vi "Auto New Vision.vi"(11 "Run?":bool) -> (2 "Side?":dbl, 3 "Done":bool)   [LabVIEW 2013]
panel:
  out "Particle Measurements (Pixels)":dbl[][](array[numeric]) format="%.2f"
  out "element":dbl
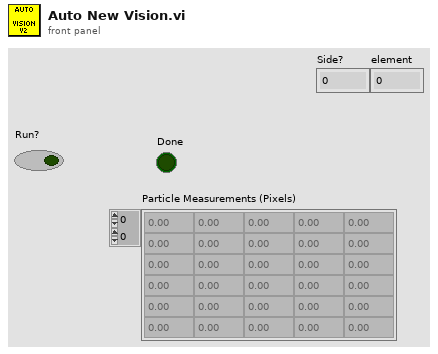
[diagram p1: front panel]
types:
  T1 = typedef "WPI_CameraDevRef.ctl" = cluster{"Camera Address":string, "CameraStatus":errorcluster, "Acquire Image Notifier":refnum<notifier>}
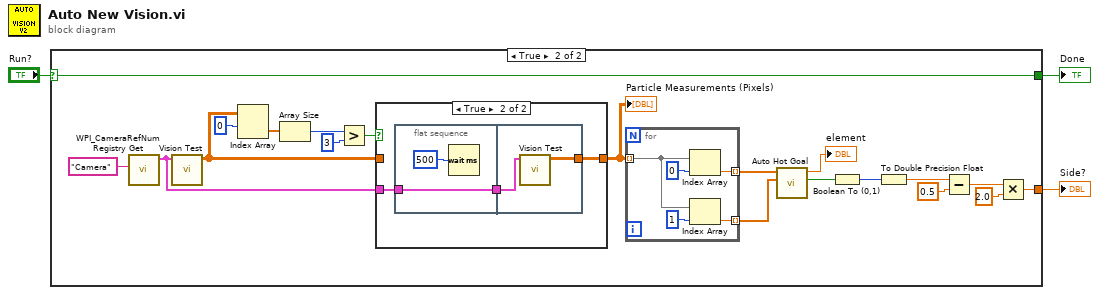
[diagram p0: block diagram]
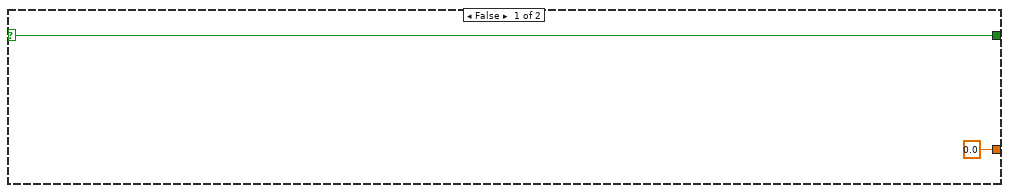
[diagram p2: hidden frame]
diagram:
  n1 = case shown="True" "Run?" {
    selector: "Run?" -> [w5 w25]
    tunnel: [w5 w25] -> w2
    tunnel: [0.0 w15] -> w1
    frame False {
    }
    frame True {
      n2 = call <vilib>:"WPI_CameraRefNum Registry Get.vi"("refnum name"="Camera") -> ("CameraDevRef"=w8:T1)  [unwired: 9 in, 1 out]
      n3 = call "Vision Test.vi"("CameraDevRef"=w8) -> ("Particle Measurements (Pixels)"=w7:dbl[][])  [unwired: 9 in, 1 out]
      n4 = Index Array(array=w7, index (row)=0 ("index")) -> (element=w12:dbl[])  [unwired: 1 in]
      n5 = Array Size(array=w12) -> (size(s)=w11:i32)
      n6 = Greater?(x=w11, y=3) -> (0:w9:bool)
      n7 = case shown="True" w9 {
        tunnel: w8 -> [_ w28]
        tunnel: w7 -> [w26 _]
        tunnel: [w26 w29] -> w6
        frame False {
        }
        frame True {
          n8 = flat-sequence {
            tunnel: w28 -> [w30]
            tunnel: [w30] -> w27
            tunnel: [w33] -> w29
            tunnel: w27 -> [w32]
            frame #0 {
              n9 = Wait (ms)(milliseconds to wait=u32 500) -> ()  [unwired: 1 out]
            }
            frame #1 {
              n10 = call "Vision Test.vi"("CameraDevRef"=w32) -> ("Particle Measurements (Pixels)"=w33:dbl[][])  [unwired: 9 in, 1 out]
            }
          }
        }
      }
      "Particle Measurements (Pixels)" <- w6
      n11 = for {
        tunnel: w6 -> [w38] mode=indexing
        tunnel: [w35] -> w24 mode=indexing
        tunnel: [w34] -> w23 mode=indexing
        n12 = Index Array(array=w38, index=0) -> (element=w35:dbl)
        n13 = Index Array(array=w38, index=1) -> (element=w34:dbl)
      }
      n14 = call "Auto Hot Goal.vi"("y"=w23, "x"=w24) -> ("x > y?"=w16:bool, "element"=→"element":dbl)  [unwired: 8 in]
      n15 = Boolean To (0,1)(Boolean=w16) -> (0, 1=w17:i16)
      n16 = To Double Precision Float(number=w17) -> (double precision float=w18:dbl)
      n17 = Subtract(x=w18, y=0.5) -> (x-y=w20:dbl)
      n18 = Multiply(x=w20, y=2.0) -> (x*y=w15:dbl)
    }
  }
  "Done" <- w2
  "Side?" <- w1
